vi "Save Data Source.vi"(0 "Database Selector":string, 1 "Driver":string, 2 "Username":string, 3 "Password":string, 4 "Schema Name":string, 5 "error in (no error)":errorcluster, 6 "Data Source Name":string, 7 "ULD FIle or Connection String":bool, 8 "Server Address":string, 9 "UDL Path":path, 10 "Port":u32, 12 "Connection String":string) -> (14 "Saved Location":path, 19 "error out (no error)":errorcluster)   [LabVIEW 2020]
uses:
  ctl/Connection Information.ctl
  <vilib>/Utility/config.llb/Write Key (String).vi
  <vilib>/Utility/config.llb/Write Key (U32).vi
  <vilib>/Utility/config.llb/Write Key (Boolean).vi
  <vilib>/Utility/config.llb/Write Key (Path).vi
  <vilib>/Utility/config.llb/NI_LVConfig.lvlib
panel:
  in  "Connection Information":T1
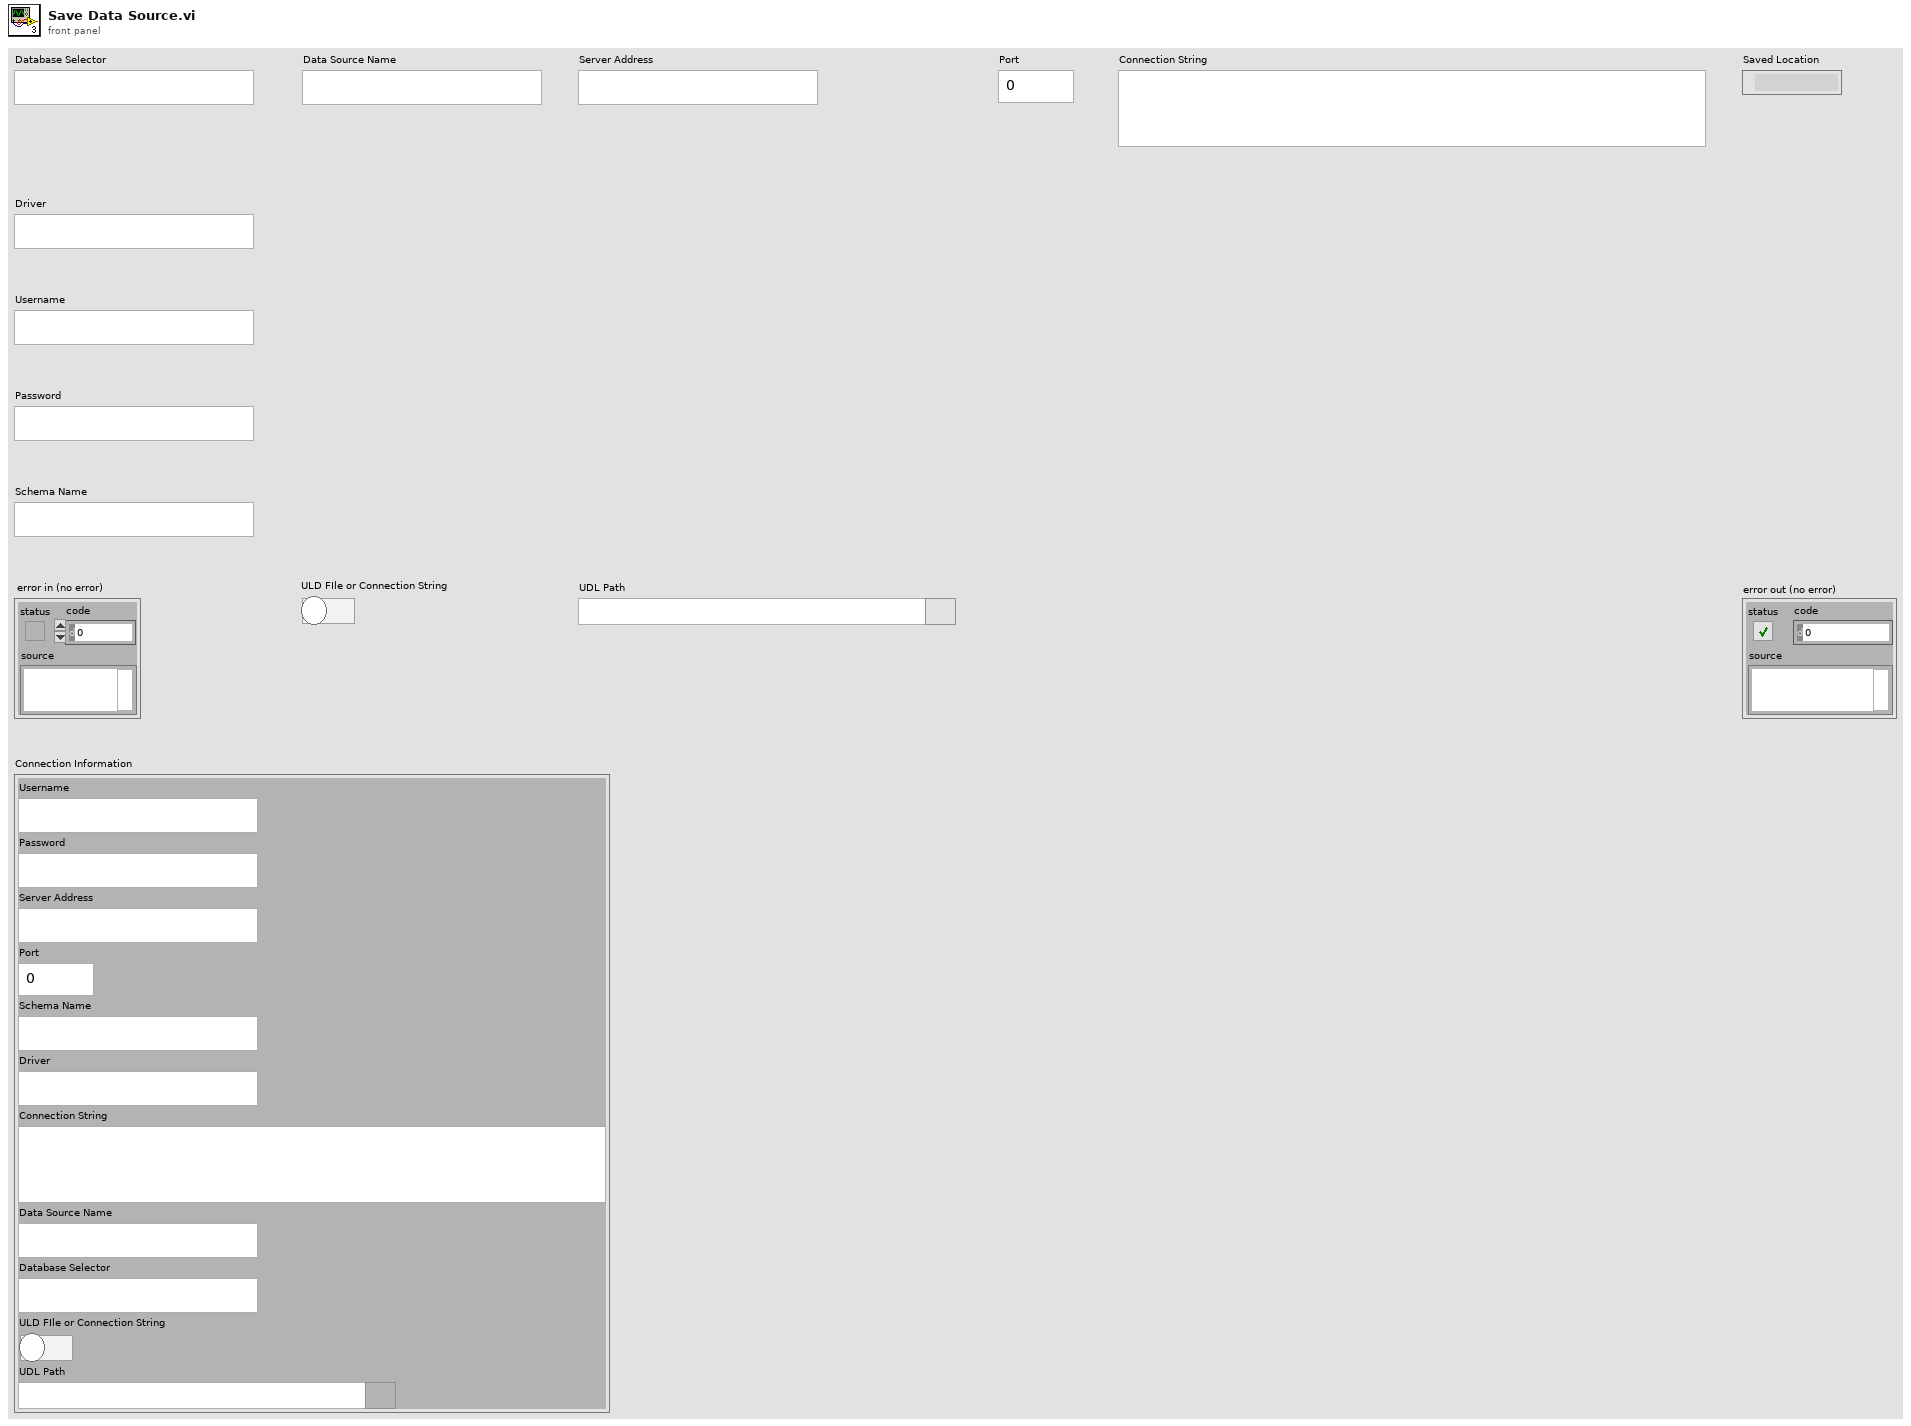
[diagram p1: front panel]
types:
  T1 = typedef "Connection Information.ctl" = cluster{"Username":string, "Password":string, "Server Address":string, "Port":u32, "Schema Name":string, "Driver":string, "Connection String":string, "Data Source Name":string, "Database Selector":string, "ULD FIle or Connection String":bool, "UDL Path":path}
  T2 = typedef "NI_LVConfig.lvlib/Config Data RefNum.ctl" = refnum<k1>
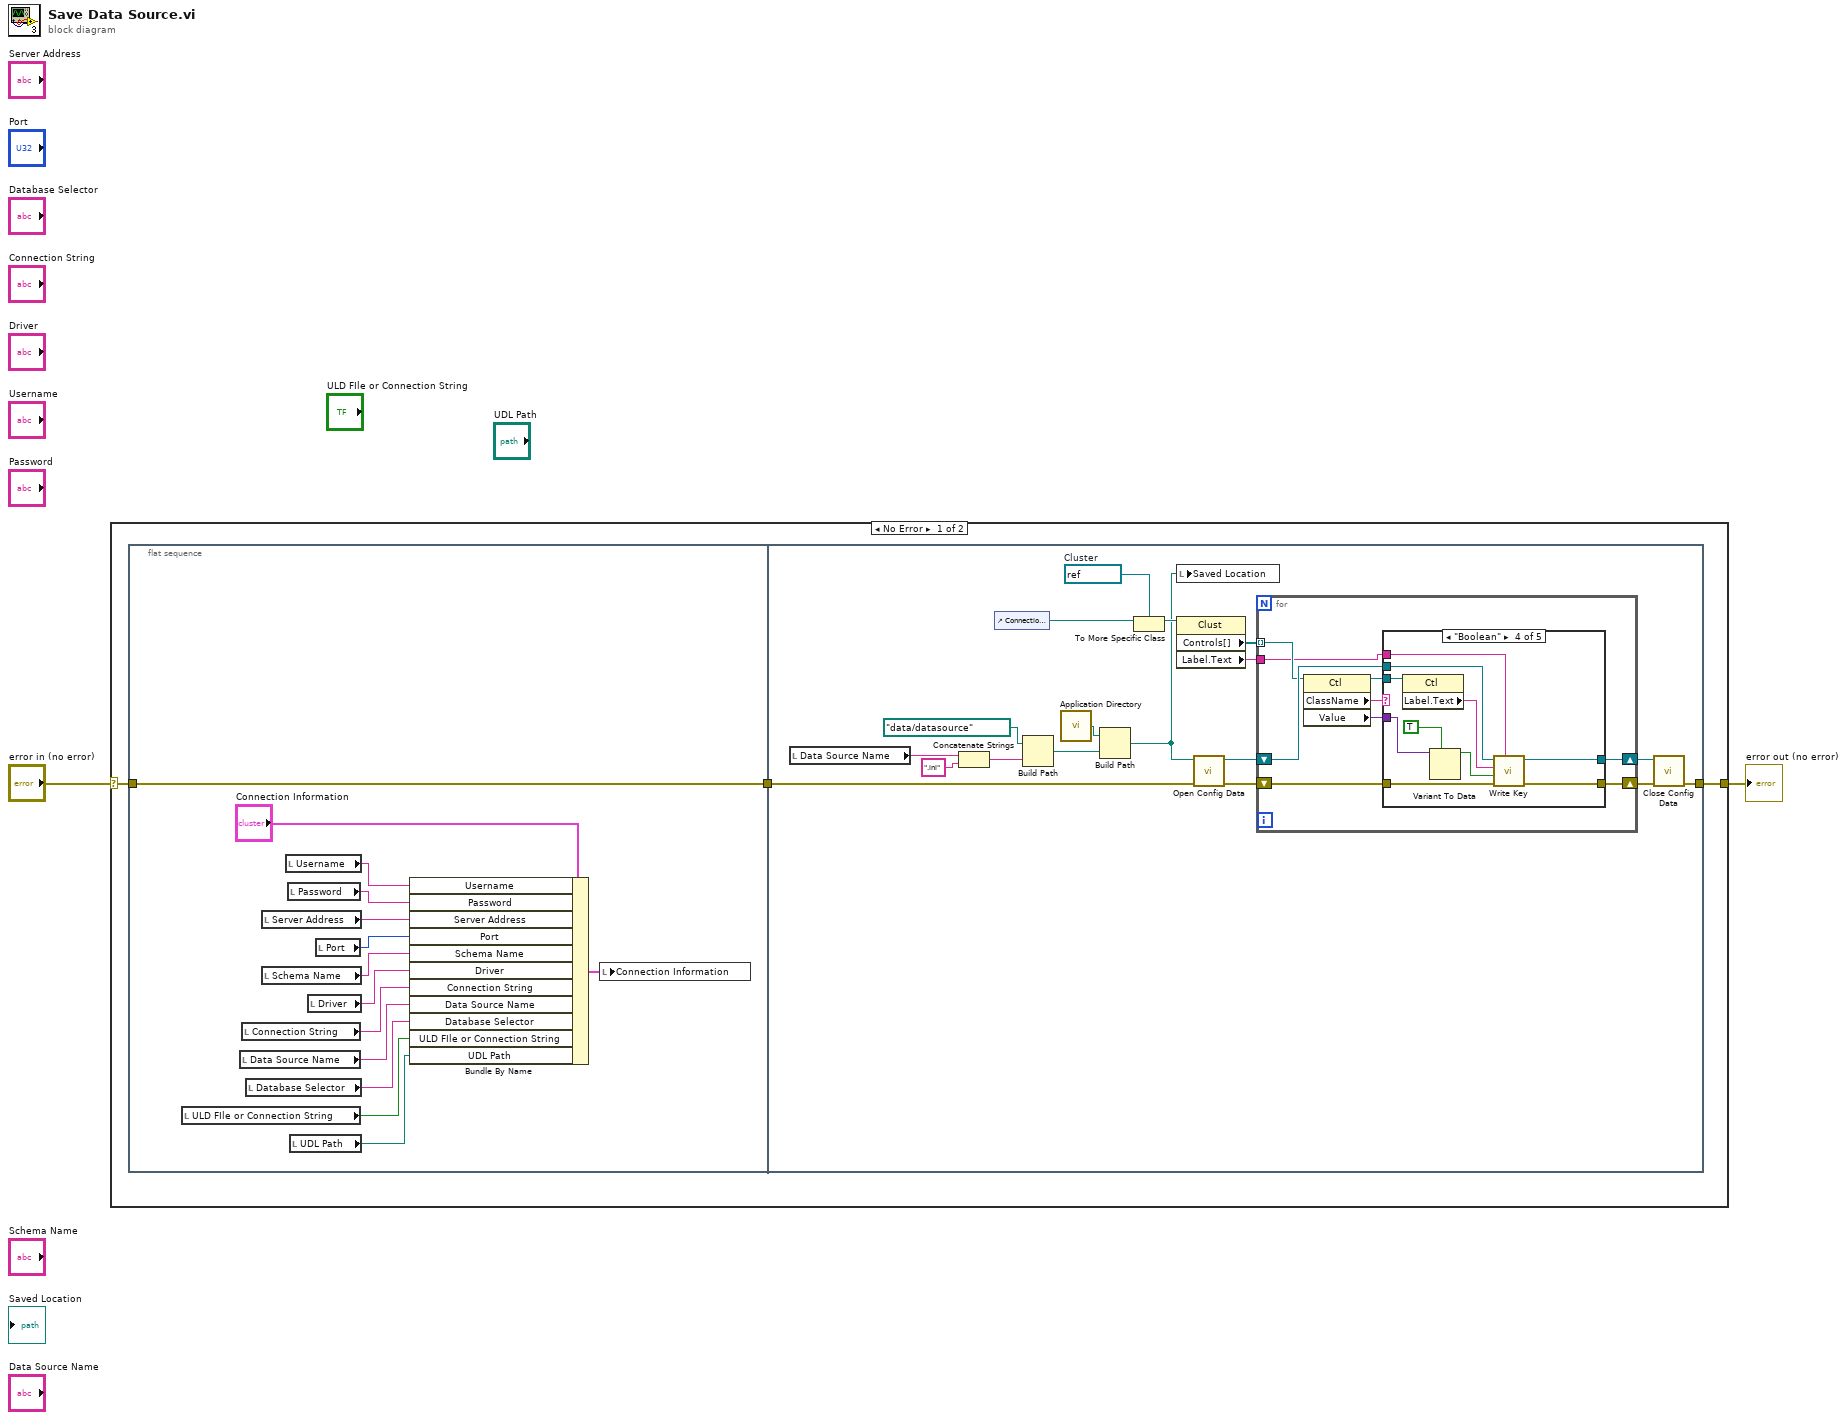
[diagram p0: block diagram]
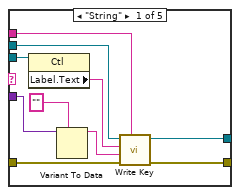
[diagram p2: hidden frame]
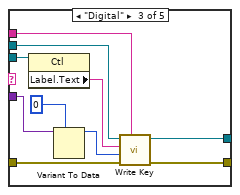
[diagram p4: hidden frame]
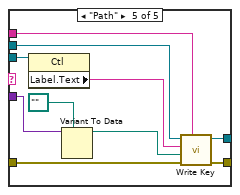
[diagram p5: hidden frame]
diagram:
  n1 = case shown="No Error" "error in (no error)" {
    selector: "error in (no error)" -> [w3 w89]
    tunnel: [w4 w89] -> w2
    frame No Error {
      n2 = flat-sequence {
        tunnel: [w9] -> w5
        tunnel: w3 -> [w9]
        tunnel: w5 -> [w25]
        tunnel: [w24] -> w4
        frame #0 {
          n3 = local read "ULD FIle or Connection String"() -> (w7:bool)
          n4 = local read "Data Source Name"() -> (w13:string)
          n5 = local read "Connection String"() -> (w10:string)
          n6 = local read "Database Selector"() -> (w11:string)
          n7 = local read "Server Address"() -> (w16:string)
          n8 = local read "Schema Name"() -> (w14:string)
          n9 = local read "Username"() -> (w18:string)
          n10 = local read "Password"() -> (w17:string)
          n11 = local read "UDL Path"() -> (w6:path)
          n12 = local read "Driver"() -> (w12:string)
          n13 = local read "Port"() -> (w15:u32)
          n14 = Bundle By Name(cluster="Connection Information", "Username"=w18, "Password"=w17, "Server Address"=w16, "Port"=w15, "Schema Name"=w14, "Driver"=w12, "Connection String"=w10, "Data Source Name"=w13, "Database Selector"=w11, "ULD FIle or Connection String"=w7, "UDL Path"=w6) -> (w8:T1)
          n15 = local write "Connection Information"(w8) -> ()
        }
        frame #1 {
          w27 = refnum<vi> refnum  # Cluster
          n16 = local read "Data Source Name"() -> (w22:string)
          n17 = Concatenate Strings(w22, ".ini" ("string")) -> (w20:string)
          n18 = control-ref of="Connection Information"() -> (w33:refnum<vi>)
          n19 = Build Path(base path=path "data/datasource" ("name or relative path"), name or relative path=w20) -> (appended path=w34:path)
          n20 = call <vilib>:"Application Directory.vi"() -> ("Application Directory"=w28:path)
          n21 = Build Path(base path=w28, name or relative path=w34) -> (appended path=w23:path)
          n22 = To More Specific Class(target class=w27, reference=w33) -> (specific class reference=w35:refnum<vi>)  [unwired: 1 in, 1 out]
          n23 = local write "Saved Location"(w23) -> ()
          n24 = property class="Clust"(reference=w35) -> ("Controls[]"=w36:refnum<vi>[], "Label.Text"=w37:string)  [unwired: 1 in, 2 out]
          n25 = call <vilib>:"Open Config Data.vi"("error in (no error)"=w25, "configuration file path"=w23) -> ("error out"=w32:errorcluster, "refnum"=w31:T2)  [unwired: 7 in, 1 out]
          n26 = for {
            tunnel: w36 -> [w40] mode=indexing
            tunnel: w37 -> [w39]
            shift-right: [w42] -> w30
            shift-left: w31 -> [w45]
            shift-right: [w41] -> w29
            shift-left: w32 -> [w44]
            n27 = property class="Ctl"(reference=w40) -> (reference out=w43:refnum<vi>, "ClassName"=w46:string, "Value"=w38:variant)  [unwired: 1 in, 1 out]
            n28 = case shown="\"Boolean\"" w46 {
              tunnel: w45 -> [w53 w58 w66 w76 w87]
              tunnel: w44 -> [w54 w57 w65 w75 w86]
              tunnel: w43 -> [w55 _ w67 w77 w88]
              tunnel: [w52 w58 w64 w74 w84] -> w42
              tunnel: [w51 w57 w63 w73 w83] -> w41
              tunnel: w39 -> [w50 _ w62 w72 w82]
              tunnel: w38 -> [w48 _ w60 w70 w80]
              frame "String" {
                n29 = property class="Ctl"(reference=w55) -> ("Label.Text"=w56:string)  [unwired: 1 in, 2 out]
                n30 = Variant To Data(type="", Variant=w48) -> (data=w47:string)  [unwired: 1 in, 1 out]
                n31 = call-poly <vilib>:"Write Key.vi"("section"=w50, "error in (no error)"=w54, "value"=w47, "key"=w56, "refnum"=w53) -> ("error out"=w51:errorcluster, "refnum out"=w52:T2)  [unwired: 4 in, 1 out]
              }
              frame "", Default {
              }
              frame "Digital" {
                n32 = property class="Ctl"(reference=w67) -> ("Label.Text"=w68:string)  [unwired: 1 in, 2 out]
                n33 = Variant To Data(type=u32 0, Variant=w60) -> (data=w59:u32)  [unwired: 1 in, 1 out]
                n34 = call-poly <vilib>:"Write Key.vi"("section"=w62, "error in (no error)"=w65, "value"=w59, "key"=w68, "refnum"=w66) -> ("error out"=w63:errorcluster, "refnum out"=w64:T2)  [unwired: 4 in, 1 out]
              }
              frame "Boolean" {
                n35 = property class="Ctl"(reference=w77) -> ("Label.Text"=w78:string)  [unwired: 1 in, 2 out]
                n36 = Variant To Data(type=TRUE, Variant=w70) -> (data=w69:bool)  [unwired: 1 in, 1 out]
                n37 = call-poly <vilib>:"Write Key.vi"("section"=w72, "error in (no error)"=w75, "value"=w69, "key"=w78, "refnum"=w76) -> ("error out"=w73:errorcluster, "refnum out"=w74:T2)  [unwired: 4 in, 1 out]
              }
              frame "Path" {
                n38 = property class="Ctl"(reference=w88) -> ("Label.Text"=w85:string)  [unwired: 1 in, 2 out]
                n39 = Variant To Data(type=path "", Variant=w80) -> (data=w79:path)  [unwired: 1 in, 1 out]
                n40 = call-poly <vilib>:"Write Key.vi"("section"=w82, "error in (no error)"=w86, "value"=w79, "key"=w85, "refnum"=w87) -> ("error out"=w83:errorcluster, "refnum out"=w84:T2)  [unwired: 4 in, 1 out]
              }
            }
          }
          n41 = call <vilib>:"Close Config Data.vi"("error in (no error)"=w29, "refnum"=w30) -> ("error out"=w24:errorcluster)  [unwired: 8 in, 1 out]
        }
      }
    }
    frame Error {
    }
  }
  "error out (no error)" <- w2
